vi "ExecuteList.vi"(1 "Element UID":u16, 2 "Speed":u16, 3 "Presence Vector":u8=2) -> (0 "Encoded JAUS Message":string)   [LabVIEW 2009]
uses:
  Support Files/Address.ctl
panel:
  in  "Destination":T1={"Subsystem Id"=90, "Node Id"=1, "Component Id"=1}
  in  "Source":T1={"Subsystem Id"=3, "Node Id"=1, "Component Id"=1}
  in  "Command Code":string="\u0004\u001c"
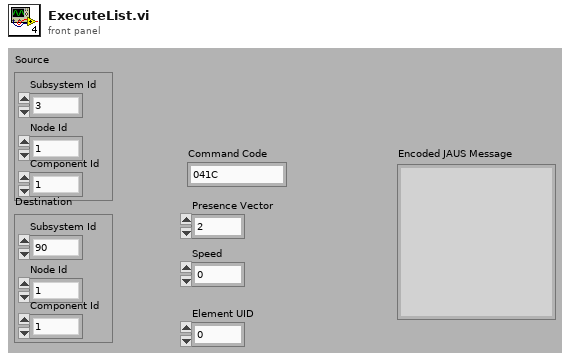
[diagram p1: front panel]
types:
  T1 = typedef "Address.ctl" = cluster{"Subsystem Id":u16, "Node Id":u8, "Component Id":u8}
  T2 = cluster{"unsigned byte array[0]":u8, "unsigned byte array[1]":u8}
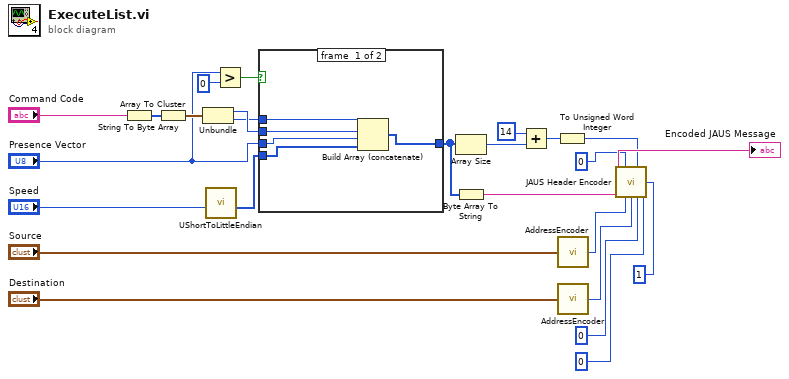
[diagram p0: block diagram]
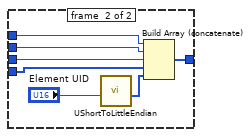
[diagram p2: hidden frame]
diagram:
  n1 = String To Byte Array(string="Command Code") -> (unsigned byte array=w13:u8[])
  n2 = Array To Cluster(array=w13) -> (cluster=w12:T2)
  n3 = Unbundle(w12) -> ("unsigned byte array[0]"=w5:u8, "unsigned byte array[1]"=w2:u8)
  n4 = call "UShortToLittleEndian.vi"("Number"="Speed") -> ("byte array"=w1:u8[])  [unwired: 10 in]
  n5 = Greater?(x="Presence Vector", y=u8 0) -> (0:w6:bool)
  n6 = case shown="True" w6 {
    tunnel: w5 -> [w29 w33]
    tunnel: "Presence Vector" -> [w28 w34]
    tunnel: [w26 w36] -> w3
    tunnel: w2 -> [w30 w32]
    tunnel: w1 -> [w27 w31]
    frame #0 {
      n7 = Build Array (concatenate)(w30, w29, w28, w27) -> (w26:u8[])
    }
    frame #1 {
      n8 = call "UShortToLittleEndian.vi"("Number"="Element UID") -> ("byte array"=w35:u8[])  [unwired: 10 in]
      n9 = Build Array (concatenate)(w32, w33, w34, w31, w35) -> (w36:u8[])
    }
  }
  n10 = Array Size(array=w3) -> (size(s)=w15:i32)
  n11 = Byte Array To String(unsigned byte array=w3) -> (string=w18:string)
  n12 = Add(x=14, y=w15) -> (x+y=w14:i32)
  n13 = To Unsigned Word Integer(number=w14) -> (unsigned 16bit integer=w9:u16)
  n14 = call "AddressEncoder.vi"("Address Cluster"="Source") -> ("Address"=w24:u32)
  n15 = call "AddressEncoder.vi"("Address Cluster"="Destination") -> ("Address"=w23:u32)
  n16 = call "JAUS Header Encoder.vi"("Message Type (0-5)"=u8 0, "Data Size (8-23)"=w9, "Priority(40-41)"=u8 1, "Payload"=w18, "Source ID (80-95)"=w24, "Destination ID (48-79)"=w23, "Data Flags (46-47)"=u8 0, "Ack/Nak (44-45)"=u8 0) -> ("Encoded JAUS Message"=→"Encoded JAUS Message":string)  [unwired: 7 in]
